vi "Check if File or Folder Exists 2.vi"(8 "error in (no error)":errorcluster, 11 "path":path) -> (0 "error out":errorcluster, 2 "file or folder exists?":bool, 3 "dup path":path)   [LabVIEW 2017]
doc: "Returns TRUE when path exists, and passes the path through. It adds error handling and tolerates an empty path, where the vi.lib version returns an error."
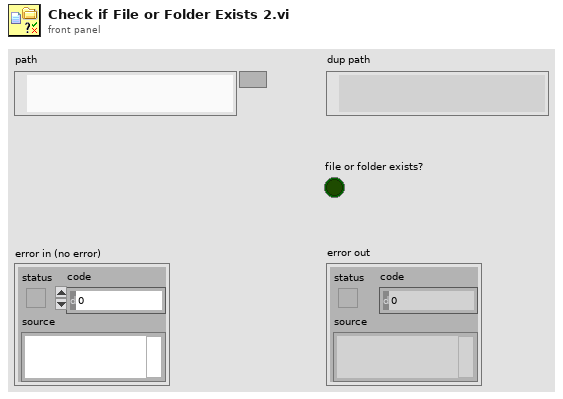
[diagram p1: front panel]
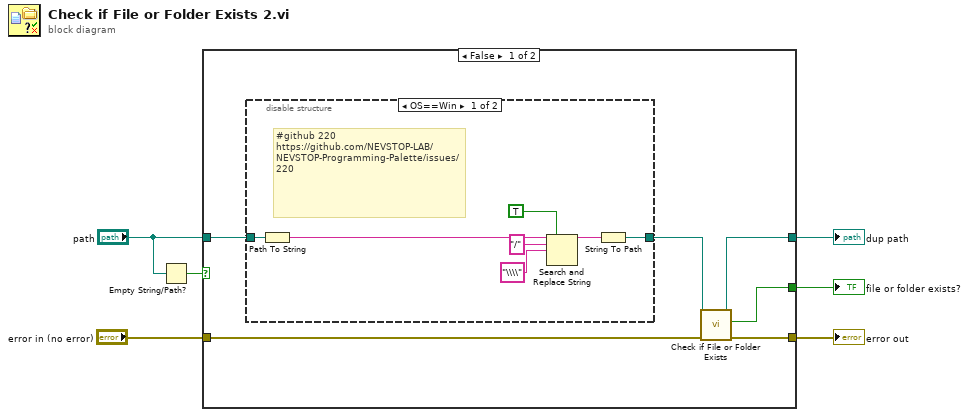
[diagram p0: block diagram]
diagram:
  n1 = Empty String/Path?(string/path="path") -> (empty?=w2:bool)
  n2 = case shown="False" w2 {
    tunnel: "error in (no error)" -> [w12 w21]
    tunnel: [w11 w21] -> w5
    tunnel: [w10 _] -> w4
    tunnel: [w9 w22] -> w3
    tunnel: "path" -> [w8 w22]
    frame False {
      n3 = disable-structure shown="OS==Win" {
        disable-tunnel: [w18 w20] -> w7
        disable-tunnel: w8 -> [w19 w20]
        frame condition #0 (active) {
          # "#github 220\nhttps://github.com/NEVSTOP-LAB/NEVSTOP-Programming-Palette/issues/220"
          n4 = Path To String(path=w19) -> (string=w16:string)
          n5 = Search and Replace String(replace all?=TRUE ("replace all? (F)"), input string=w16, search string="/", replace string="\\\\" ("search string")) -> (result string=w17:string)  [unwired: 4 in, 3 out]
          n6 = String To Path(string=w17) -> (path=w18:path)
        }
        frame condition #1 {
        }
      }
      n7 = call <vilib>:"Check if File or Folder Exists.vi"("error in (no error)"=w12, "path"=w7) -> ("error out"=w11:errorcluster, "file or folder exists?"=w10:bool, "dup path"=w9:path)  [unwired: 7 in]
    }
    frame True {
    }
  }
  "error out" <- w5
  "file or folder exists?" <- w4
  "dup path" <- w3
